vi "GPS Parsing.vi"() -> (0 "GPS error out":errorcluster caption="error out")   [LabVIEW 2016]
panel:
  in  "stop?":bool
  in  "GPS error in":errorcluster
  in  "GPS Baud rate":u32(ring)=38400 items=["Auto Connect"=0, "300"=300, "600"=600, "1200"=1200, "2400"=2400, "4800"=4800, "9600"=9600, "19200"=19200, "38400"=38400, "57600"=57600, "115200"=115200]
  out "GPS port out":refnum<visa-resource-name>
  out "Time":string
  out "N/S":string
  out "E/W":string
  out "Chechsum 부분":string
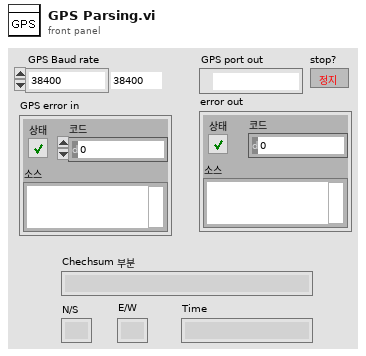
[diagram p1: front panel]
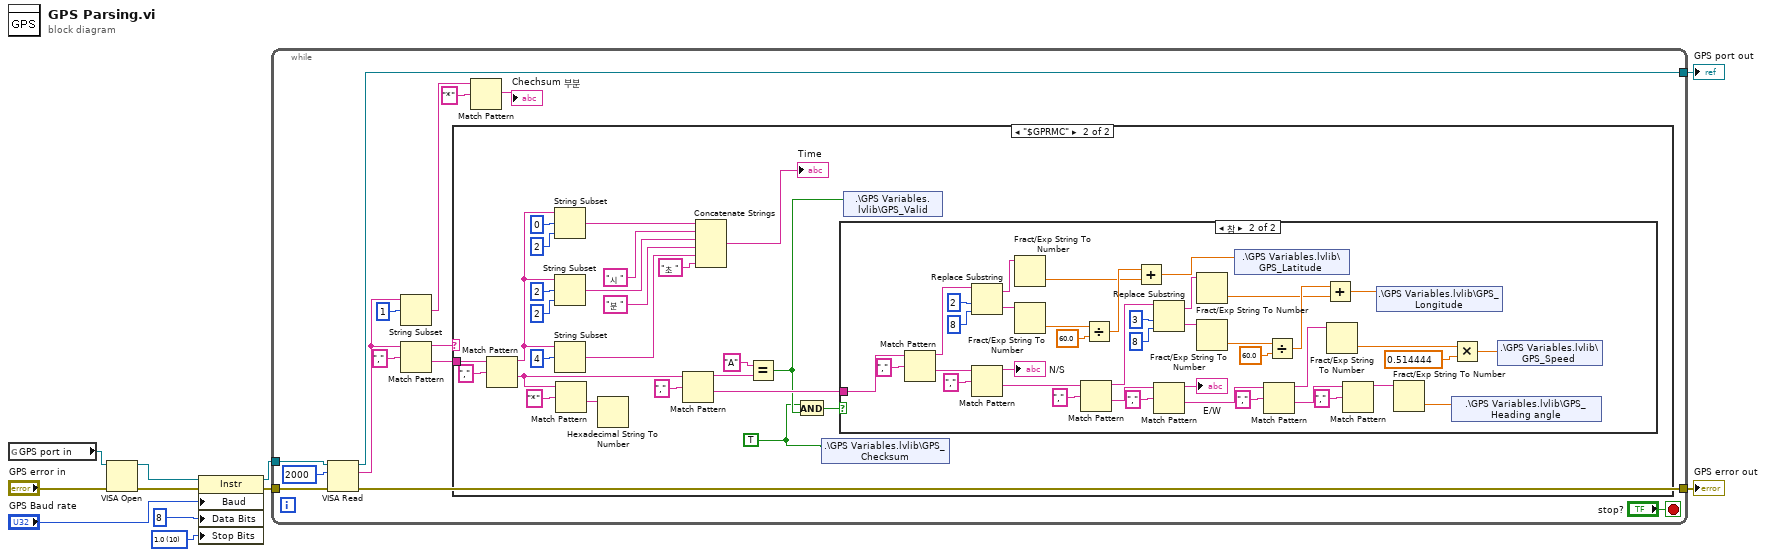
[diagram p0: block diagram]
diagram:
  w8 = u16 10 items=["1.0"=10, "1.5"=15, "2.0"=20] ("Serial Settings:Stop Bits")
  n1 = global read "[GV]_GPS Port NUM.vi" "GPS port in"() -> (w1:refnum<visa-resource-name>)
  n2 = VISA Open(error in (no error)="GPS error in", VISA resource name=w1) -> (VISA resource name=w2:refnum<visa-resource-name>, error out=w6:errorcluster)  [unwired: 3 in]
  n3 = property class="Instr"(reference=w2, error in=w6, "Baud"="GPS Baud rate", "Data Bits"=u16 8 ("Serial Settings:Data Bits"), "Stop Bits"=w8) -> (reference out=w4:refnum<visa-resource-name>, error out=w3:errorcluster)
  n4 = while {
    tunnel: w4 -> [w17]
    tunnel: w3 -> [w16]
    tunnel: [w14] -> w10
    tunnel: [w13] -> w11
    stop <- "stop?" stop-if-true
    n5 = VISA Read(VISA resource name=w17, byte count=u32 2000 ("바이트 카운트"), error in (no error)=w16) -> (VISA resource name out=w14:refnum<visa-resource-name>, read buffer=w18:string, error out=w13:errorcluster)  [unwired: 1 out]
    n6 = String Subset(string=w18, offset (0)=1 ("오프셋(0)")) -> (substring=w19:string)  [unwired: 1 in]
    n7 = Match Pattern(string=w18, regular expression="," ("정규식")) -> (before substring=w24:string, after substring=w23:string)  [unwired: 1 in, 2 out]
    n8 = case shown="\"$GPRMC\"" w24 {
      tunnel: w23 -> [_ w49]
      frame "거짓", Default {
      }
      frame "$GPRMC" {
        w26 = TRUE ("x")
        n9 = Match Pattern(string=w49, regular expression="," ("정규식")) -> (before substring=w34:string, after substring=w31:string)  [unwired: 1 in, 2 out]
        n10 = String Subset(string=w34, offset (0)=0 ("오프셋(0)"), length (rest)=2 ("길이(나머지)")) -> (substring=w40:string)
        n11 = String Subset(string=w34, offset (0)=2 ("오프셋(0)"), length (rest)=2 ("길이(나머지)")) -> (substring=w43:string)
        n12 = String Subset(string=w34, offset (0)=4 ("오프셋(0)")) -> (substring=w46:string)  [unwired: 1 in]
        n13 = Match Pattern(string=w31, regular expression="*" ("정규식")) -> (after substring=w30:string)  [unwired: 1 in, 3 out]
        n14 = Hexadecimal String To Number(string=w30) -> ()  [unwired: 2 in, 2 out]
        n15 = Match Pattern(string=w31, regular expression="," ("정규식")) -> (before substring=w33:string, after substring=w28:string)  [unwired: 1 in, 2 out]
        n16 = Concatenate Strings(w40, "시 ", w43, "분 ", w46, "초 ") -> (→"Time":string)
        n17 = Equal?(x="A" ("y"), y=w33) -> (x = y?=w27:bool)
        n18 = And(x=w26, y=w27) -> (x .and. y?=w29:bool)
        n19 = shared-variable ".\\GPS Variables.lvlib\\GPS_Checksum"(w26) -> ()  [unwired: 1 in, 1 out]
        n20 = case shown="참" w29 {
          tunnel: w28 -> [_ w90]
          frame False {
          }
          frame True {
            n21 = Match Pattern(string=w90, regular expression="," ("정규식")) -> (before substring=w72:string, after substring=w71:string)  [unwired: 1 in, 2 out]
            n22 = Replace Substring(2:8 ("위도_길이(부분 문자열의 길이)"), 3:2 ("위도_오프셋"), 5:w72) -> (0:w84:string, 1:w83:string)  [unwired: 1 in]
            n23 = Match Pattern(string=w71, regular expression="," ("정규식")) -> (before substring=→"N/S":string, after substring=w68:string)  [unwired: 1 in, 2 out]
            n24 = Fract/Exp String To Number(string=w83) -> (number=w81:dbl)  [unwired: 1 in, 3 out]
            n25 = Fract/Exp String To Number(string=w84) -> (number=w85:dbl)  [unwired: 1 in, 3 out]
            n26 = Match Pattern(string=w68, regular expression="," ("정규식")) -> (before substring=w67:string, after substring=w64:string)  [unwired: 1 in, 2 out]
            n27 = Divide(x=w85, y=60.0) -> (x/y=w82:dbl)
            n28 = Add(x=w82, y=w81) -> (x+y=w53:dbl)
            n29 = Replace Substring(2:8 ("경도_길이(부분 문자열의 길이)"), 3:3 ("경도_오프셋(0)"), 5:w67) -> (0:w77:string, 1:w76:string)  [unwired: 1 in]
            n30 = Match Pattern(string=w64, regular expression="," ("정규식")) -> (before substring=→"E/W":string, after substring=w61:string)  [unwired: 1 in, 2 out]
            n31 = Fract/Exp String To Number(string=w76) -> (number=w74:dbl)  [unwired: 4 out]
            n32 = Fract/Exp String To Number(string=w77) -> (number=w66:dbl)  [unwired: 4 out]
            n33 = shared-variable ".\\GPS Variables.lvlib\\GPS_Latitude"(w53) -> ()  [unwired: 1 in, 1 out]
            n34 = Match Pattern(string=w61, regular expression="," ("정규식")) -> (before substring=w58:string, after substring=w56:string)  [unwired: 1 in, 2 out]
            n35 = Divide(x=w66, y=60.0) -> (x/y=w75:dbl)
            n36 = Add(x=w75, y=w74) -> (x+y=w52:dbl)
            n37 = Fract/Exp String To Number(string=w58) -> (number=w59:dbl)  [unwired: 3 in, 1 out]
            n38 = Match Pattern(string=w56, regular expression="," ("정규식")) -> (before substring=w55:string)  [unwired: 1 in, 3 out]
            n39 = shared-variable ".\\GPS Variables.lvlib\\GPS_Longitude"(w52) -> ()  [unwired: 1 in, 1 out]
            n40 = Fract/Exp String To Number(string=w55) -> (number=w54:dbl)  [unwired: 3 in, 1 out]
            n41 = Multiply(x=w59, y=0.514444) -> (x*y=w51:dbl)
            n42 = shared-variable ".\\GPS Variables.lvlib\\GPS_Heading angle"(w54) -> ()  [unwired: 1 in, 1 out]
            n43 = shared-variable ".\\GPS Variables.lvlib\\GPS_Speed"(w51) -> ()  [unwired: 1 in, 1 out]
          }
        }
        n44 = shared-variable ".\\GPS Variables.lvlib\\GPS_Valid"(w27) -> ()  [unwired: 1 in, 1 out]
      }
    }
    n45 = Match Pattern(string=w19, regular expression="*" ("정규식")) -> (before substring=→"Chechsum 부분":string)  [unwired: 1 in, 3 out]
  }
  "GPS error out" <- w11
  "GPS port out" <- w10
